vi "Initialize Data Channels.vi"(8 "error in (no error)":errorcluster, 10 "Framework Configuration":refnum<class "Framework Configuration.lvclass">, 11 "VeriStand Data Sharing Framework in":refnum<class "VeriStand DSF.lvclass">) -> (0 "error out":errorcluster, 1 "data channels refs":T1[](array[typedef]) format="%.0x", 2 "data channel offsets":u64[](array[numeric]) format="%.0x", 3 "VeriStand Data Sharing Framework out":refnum<class "VeriStand DSF.lvclass">)   [LabVIEW 2017, in "DSF Engine.lvlib" / "VeriStand DSF.lvclass"]
uses:
  VeriStand DSF.lvclass
  DSF Core.lvlibp/Classes/Configuration/Core/Framework/Framework Configuration.lvclass
  <vilib>/NI Veristand/Custom Device API/Custom Device Item Ref.ctl
  VeriStand DSF.lvclass/VeriStand DSF.ctl
  <vilib>/NI Veristand/Custom Device API/Data Access Type.ctl
  DSF Core.lvlibp/Typedefs/DSF Direction.ctl
  Shared/Data Channel Page GUID.vi
  <vilib>/NI Veristand/Custom Device API/Custom Device API.lvlib
  DSF Core.lvlibp
  Shared/DSF Shared.lvlib
  DSF Core.lvlibp/Classes/Configuration/Core/Thread/Thread Configuration.lvclass
  DSF Core.lvlibp/Classes/Configuration/Core/Plugin/Plugin Configuration.lvclass
  DSF Core.lvlibp/Classes/Configuration/Core/Group/Group Configuration.lvclass
  DSF Core.lvlibp/Classes/Configuration/Core/Transfer/Transfer Configuration.lvclass
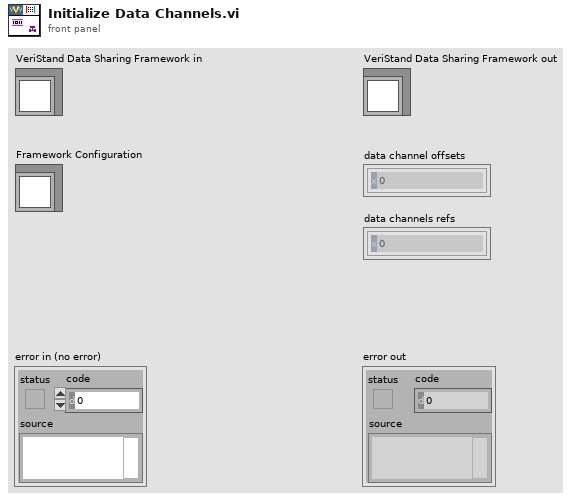
[diagram p1: front panel]
types:
  T1 = typedef "Custom Device API.lvlib/Custom Device Item Ref.ctl" = u64
  T2 = typedef "Custom Device API.lvlib/Data Access Type.ctl" = enum16{"Read", "Write"}
  T3 = typedef "DSF Core.lvlibp/DSF Direction.ctl" = enum8{"Tx", "Rx"}
  T4 = typedef "DSF Core.lvlibp/Group Configuration.lvclass/Core Group Configuration.ctl" = cluster{"name":string, "direction":T3, "cycle timing":T5, "timeout behavior":T6, "enable conversion":bool}
  T5 = typedef "DSF Core.lvlibp/DSF Timing Info.ctl" = cluster{"priority":u64, "decimation":u64, "offset":u64}
  T6 = typedef "DSF Core.lvlibp/DSF Timeout Behavior.ctl" = enum8{"Increment Late Count", "Throw Error"}
  T7 = typedef "DSF Core.lvlibp/Transfer Configuration.lvclass/Channel Configuration.ctl" = cluster{"configuration":T8, "component settings":T10[]}
  T8 = typedef "DSF Core.lvlibp/Channel Configuration.lvclass/Core Channel Configuration.ctl" = cluster{"name":string, "units":string, "engine data type":T9, "string data type":T9, "string offset":u64}
  T9 = typedef "DSF Core.lvlibp/DSF Data Type.ctl" = enum8{"Bool", "SGL", "DBL", "I8", "I16", "I32", "I64", "U8", "U16", "U32", "U64"}
  T10 = typedef "DSF Core.lvlibp/DSF Settings Info.ctl" = cluster{"component":string, "values":cluster{"key":string, "value":string}[]}
  T11 = typedef "Custom Device API.lvlib/Data Reference.ctl" = i32
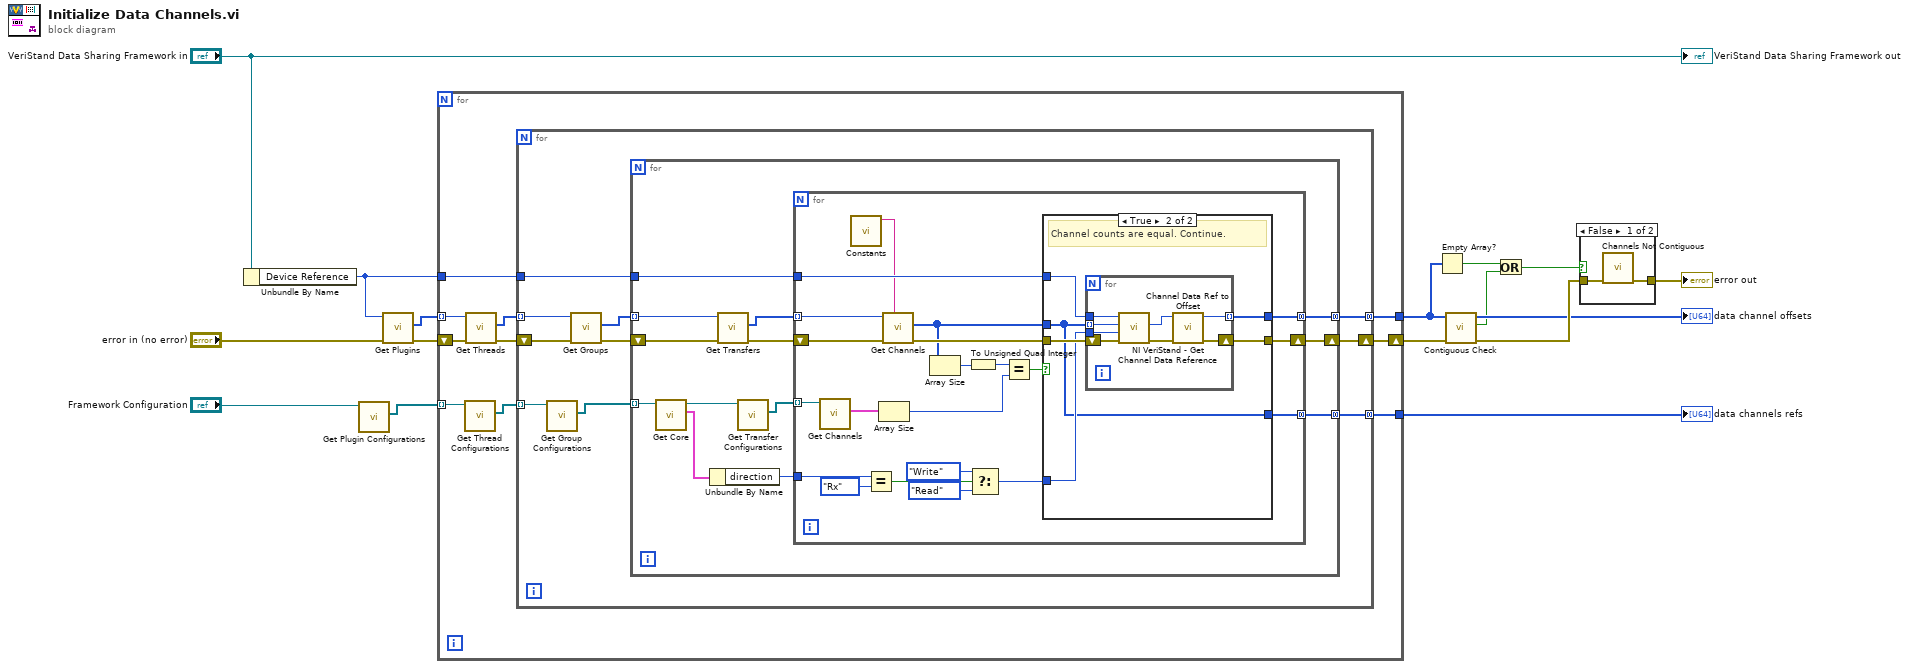
[diagram p0: block diagram]
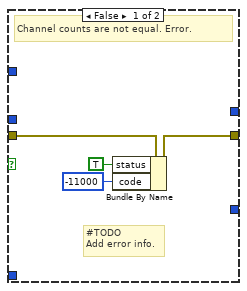
[diagram p2: hidden frame]
diagram:
  n1 = Unbundle By Name("VeriStand Data Sharing Framework in") -> ("Device Reference"=w12:T1)
  n2 = call "Get Plugin Configurations.vi"("Framework Configuration in"="Framework Configuration") -> ("Plugin Configurations"=w2:refnum<class "Plugin Configuration.lvclass">[])  [unwired: 8 in, 2 out]
  n3 = call "Get Plugins.vi"("error in (no error)"="error in (no error)", "Item Ref in"=w12) -> ("error out"=w15:errorcluster, "Plugin refs"=w14:T1[])  [unwired: 7 in, 1 out]
  n4 = for {
    tunnel: w14 -> [w21] mode=indexing
    tunnel: w12 -> [w25]
    tunnel: [w24] -> w9
    tunnel: [w23] -> w8
    tunnel: w2 -> [w18] mode=indexing
    shift-right: [w26] -> w16
    shift-left: w15 -> [w22]
    n5 = call "Get Thread Configurations.vi"("Plugin Configuration in"=w18) -> ("Thread Configurations"=w17:refnum<class "Thread Configuration.lvclass">[])  [unwired: 8 in, 2 out]
    n6 = call "Get Threads.vi"("error in (no error)"=w22, "Item Ref in"=w21) -> ("error out"=w20:errorcluster, "Plugin refs"=w19:T1[])  [unwired: 7 in, 1 out]
    n7 = for {
      tunnel: w19 -> [w32] mode=indexing
      tunnel: w17 -> [w28] mode=indexing
      tunnel: w25 -> [w36]
      shift-right: [w35] -> w26
      shift-left: w20 -> [w33]
      tunnel: [w34] -> w23 mode=concatenating
      tunnel: [w29] -> w24 mode=concatenating
      n8 = call "Get Group Configurations.vi"("Thread Configuration in"=w28) -> ("Group Configurations"=w27:refnum<class "Group Configuration.lvclass">[])  [unwired: 8 in, 2 out]
      n9 = call "Get Groups.vi"("error in (no error)"=w33, "Plugin Ref in"=w32) -> ("error out"=w31:errorcluster, "Group refs"=w30:T1[])  [unwired: 7 in, 1 out]
      n10 = for {
        tunnel: w27 -> [w41] mode=indexing
        tunnel: w30 -> [w45] mode=indexing
        tunnel: w36 -> [w49]
        shift-right: [w48] -> w35
        shift-left: w31 -> [w46]
        tunnel: [w47] -> w34 mode=concatenating
        tunnel: [w42] -> w29 mode=concatenating
        n11 = call "Get Core.vi"("Group Configuration in"=w41) -> ("core"=w37:T4, "Group Configuration out"=w40:refnum<class "Group Configuration.lvclass">)  [unwired: 8 in, 1 out]
        n12 = Unbundle By Name(w37) -> ("direction"=w38:T3)
        n13 = call "Get Transfers.vi"("error in (no error)"=w46, "Group Ref in"=w45) -> ("error out"=w44:errorcluster, "Transfer refs"=w43:T1[])  [unwired: 7 in, 1 out]
        n14 = call "Get Transfer Configurations.vi"("Group Configuration in"=w40) -> ("Transfer Configurations"=w39:refnum<class "Transfer Configuration.lvclass">[])  [unwired: 8 in, 2 out]
        n15 = for {
          tunnel: w39 -> [w52] mode=indexing
          tunnel: w43 -> [w59] mode=indexing
          tunnel: w49 -> [w63]
          shift-right: [w61] -> w48
          shift-left: w44 -> [w53]
          tunnel: [w60] -> w47 mode=concatenating
          tunnel: [w56] -> w42 mode=concatenating
          tunnel: w38 -> [w54]
          n16 = call "Get Channels.vi"("Transfer Configuration in"=w52) -> ("channels"=w51:T7[])  [unwired: 8 in, 2 out]
          n17 = call-poly "Constants.vi"() -> ("Status GUID"=w55:string)  [unwired: 11 in]
          n18 = Equal?(x=w54, y=DSF_Direction."Rx") -> (x = y?=w68:bool)
          n19 = Array Size(array=w51) -> (size(s)=w50:i32)
          n20 = call "Get Channels.vi"("GUID (Default Channel)"=w55, "error in (no error)"=w53, "Item Ref in"=w59) -> ("error out"=w58:errorcluster, "Channels refs"=w57:T1[])  [unwired: 6 in, 1 out]
          n21 = Array Size(array=w57) -> (size(s)=w70:i32)
          n22 = To Unsigned Quad Integer(1:w70) -> (0:w64:u64)
          n23 = Select(t=Data_Access_Type."Write" ("Access"), s=w68, f=Data_Access_Type."Read") -> (s? t:f=w62:T2)
          n24 = Equal?(x=w64, y=w50) -> (x = y?=w65:bool)
          n25 = case shown="True" w65 {
            tunnel: w57 -> [_ w75]
            tunnel: w63 -> [_ w79]
            tunnel: w62 -> [_ w78]
            tunnel: w58 -> [w74 w80]
            tunnel: [w73 w76] -> w61
            tunnel: [_ w77] -> w60
            tunnel: [_ w75] -> w56
            frame False {
              # "#TODO\nAdd error info."
              # "Channel counts are not equal. Error."
              n26 = Bundle By Name(cluster=w74, "status"=TRUE, "code"=-11000) -> (w73:errorcluster)
            }
            frame True {
              # "Channel counts are equal. Continue."
              n27 = for {
                tunnel: w79 -> [w87]
                tunnel: w78 -> [w86]
                tunnel: w75 -> [w85] mode=indexing
                tunnel: [w81] -> w77 mode=indexing
                shift-right: [w82] -> w76
                shift-left: w80 -> [w88]
                n28 = call <vilib>:"NI VeriStand - Get Channel Data Reference.vi"("error in (no error)"=w88, "Access"=w86, "Channel Ref in"=w85, "Device Ref in"=w87) -> ("error out"=w84:errorcluster, "Channel Data Reference"=w83:T11)  [unwired: 5 in, 1 out]
                n29 = call "Channel Data Ref to Offset.vi"("error in (no error)"=w84, "Channel Data Reference"=w83) -> ("error out"=w82:errorcluster, "channel offset"=w81:u64)  [unwired: 8 in]
              }
            }
          }
        }
      }
    }
  }
  "data channels refs" <- w9
  n30 = Empty Array?(array=w8) -> (empty?=w7:bool)
  n31 = call "Contiguous Check.vi"("error in (no error)"=w16, "channel offsets in"=w8) -> ("error out"=w11:errorcluster, "contiguous?"=w4:bool, "channel offsets out"=→"data channel offsets":u64[])  [unwired: 7 in]
  n32 = Or(x=w7, y=w4) -> (x .or. y?=w6:bool)
  n33 = case shown="False" w6 {
    tunnel: [w90 w91] -> w10
    tunnel: w11 -> [w89 w91]
    frame False {
      n34 = call "Channels Not Contiguous.vi"("error in (no error)"=w89) -> ("error out"=w90:errorcluster)  [unwired: 10 in]
    }
    frame True {
    }
  }
  "error out" <- w10
  "VeriStand Data Sharing Framework out" <- "VeriStand Data Sharing Framework in"
